vi "myRIO v1.0 Config Timer IRQ.vi"(6 "Remaining Time":u32, 7 "Timer ID":u8, 8 "error in (no error)":errorcluster, 9 "Action":enum16{"Add", "Update", "Remove"}(ring), 11 "myRIO FPGA Ref In":T2) -> (0 "error out":errorcluster, 1 "Timer IDs":u8[](array[numeric]), 3 "Callback VI Refs":T1[](array[typedef]))   [LabVIEW 2021]
uses:
  <vilib>/myRIO/Common/Instrument Driver Framework/Utilities/typedefs/Generic FPGA Reference.ctl
  <vilib>/myRIO/Common/Instrument Driver Framework/myRIO v1.0/IRQ/typedefs/Callback VI Ref.ctl
  <vilib>/myRIO/Common/Instrument Driver Framework/myRIO v1.0/IRQ/typedefs/Timer IRQ FPGA Reference.ctl
  <vilib>/myRIO/Common/Instrument Driver Framework/Utilities/typedefs/FPGA Ref Manager Action Enum.ctl
  <vilib>/Utility/error.llb/Error Cluster From Error Code.vi
  <vilib>/rvi/errors/niLvFpgaAdjustHostInterfaceError.vi
  <vilib>/rvi/interface/nirviReadWriteControl/nirviReadWriteControl.xnode
  <vilib>/rvi/interface/Simulation/niFpgaSimulationCallBeginRW.vi
  NiFpgaLv.dll
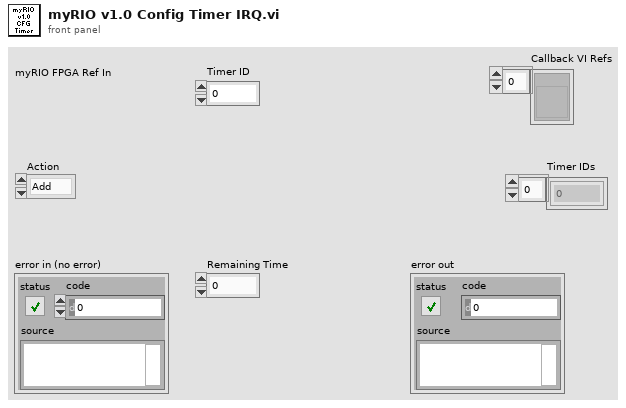
[diagram p1: front panel]
types:
  T1 = typedef "Callback VI Ref.ctl" = refnum<vi>
  T2 = typedef "Generic FPGA Reference.ctl" = refnum<k20>
  T3 = typedef "FPGA Ref Manager Action Enum.ctl" = enum16{"Get", "Set", "Reset"}
  T4 = typedef "Timer IRQ FPGA Reference.ctl" = refnum<k20>
  T5 = typedef "Timer IRQ Array.ctl" = T6[]
  T6 = typedef "Timer IRQ.ctl" = cluster{"Remaining(us)":u32, "Timer ID":u8, "Interval(us)":u32, "Callback VI Ref":T1, "Allow Overwrite?":bool, "Timer enabled?":bool}
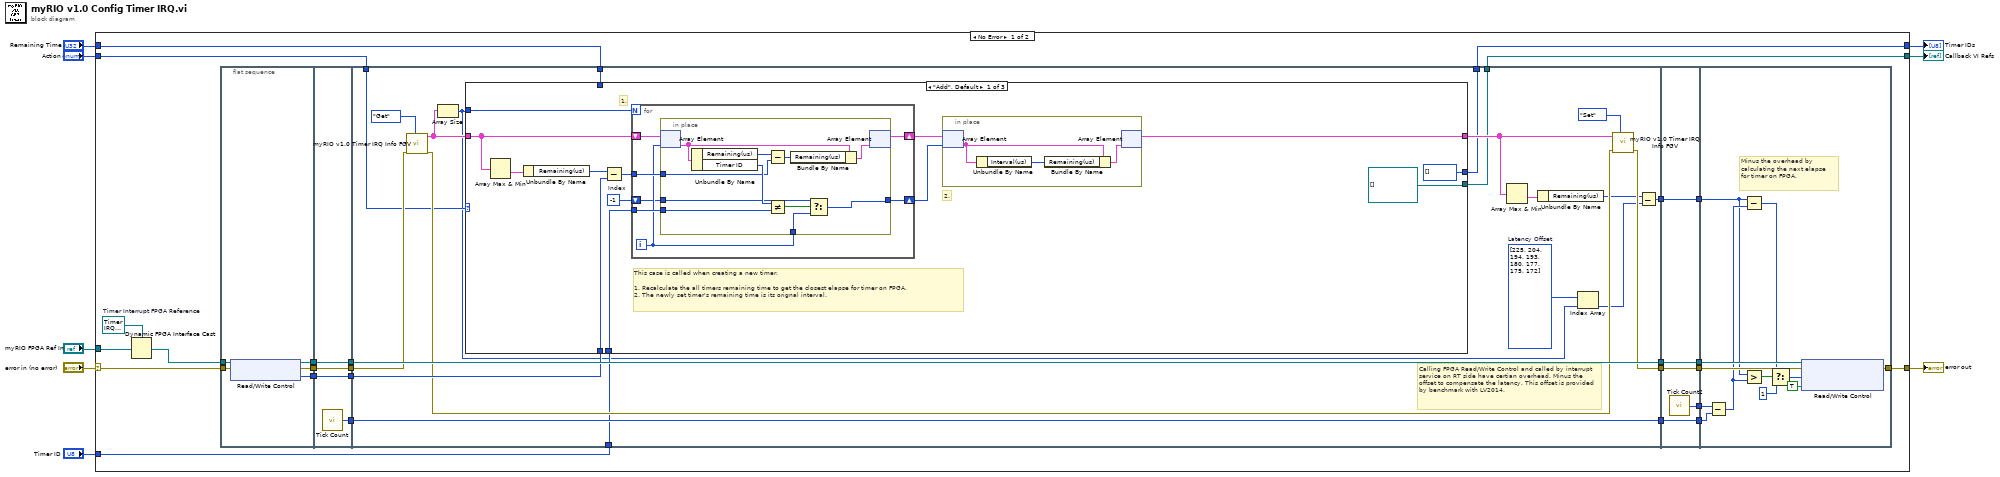
[diagram p0: block diagram]
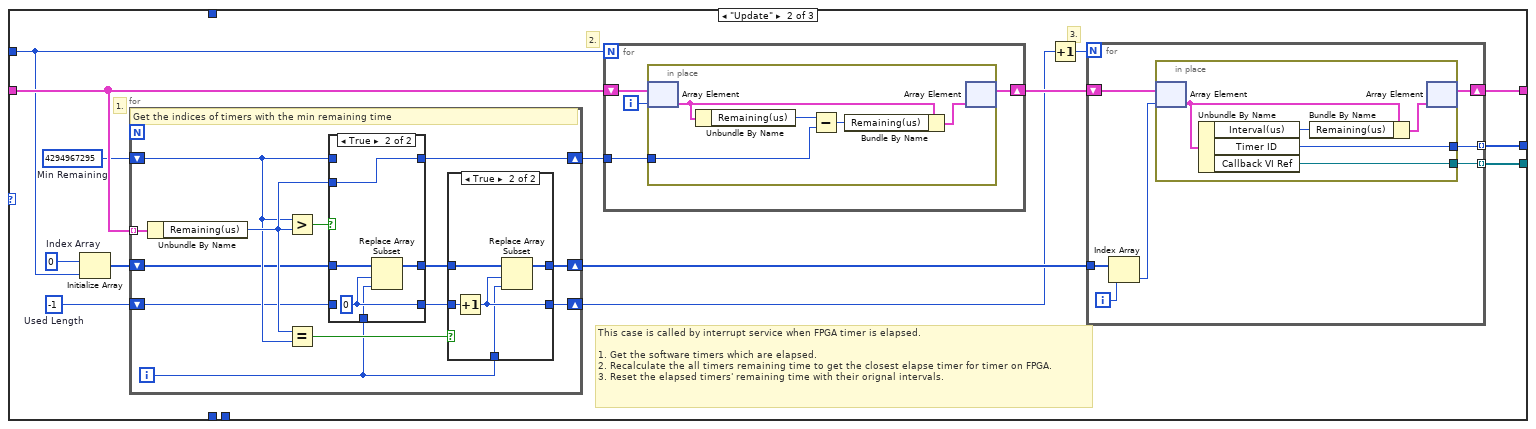
[diagram p2: hidden frame]
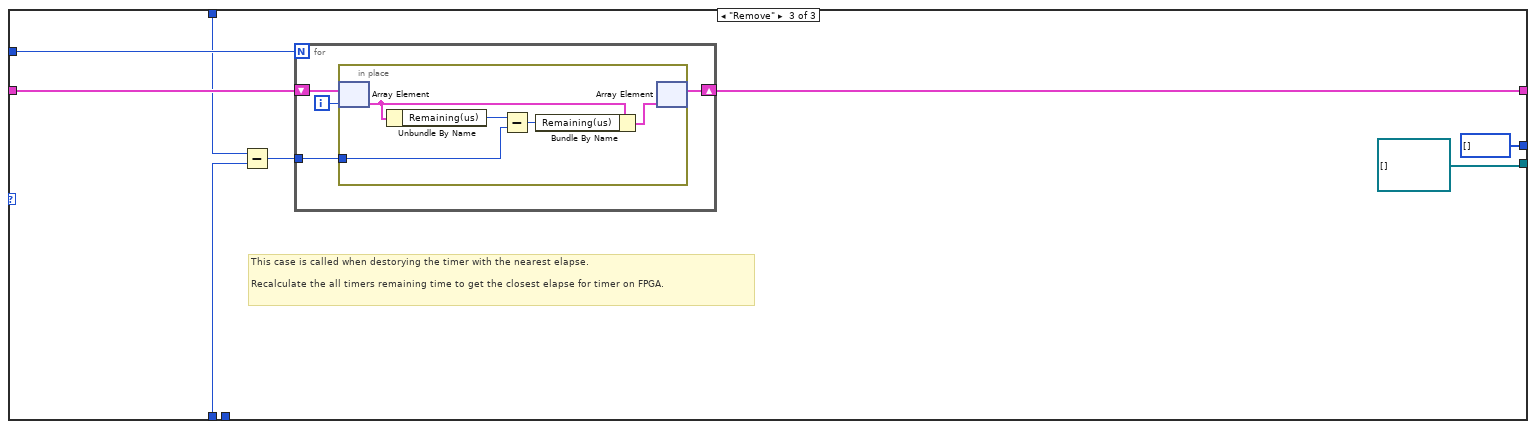
[diagram p5: hidden frame]
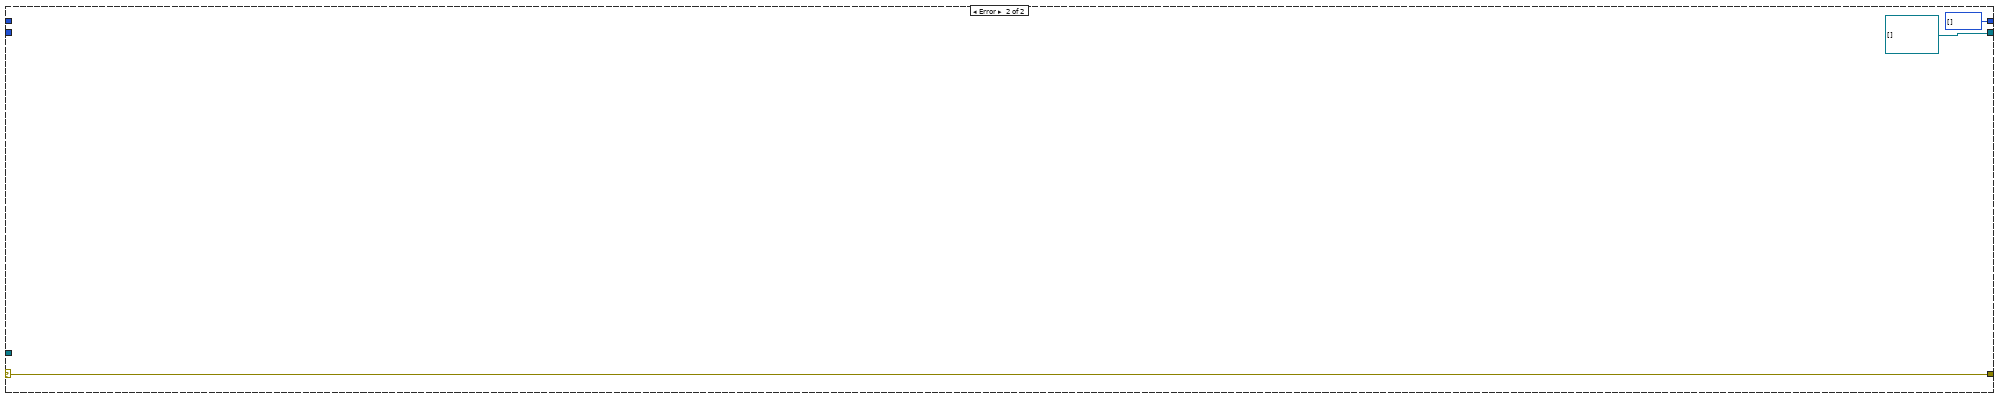
[diagram p6: hidden frame]
diagram:
  n1 = case shown="No Error" "error in (no error)" {
    selector: "error in (no error)" -> [w31 w198]
    tunnel: [w22 w198] -> w8
    tunnel: "myRIO FPGA Ref In" -> [w33 _]
    tunnel: "Timer ID" -> [w10 _]
    tunnel: [w13 T1[] []] -> w3
    tunnel: [w12 u8[] []] -> w4
    tunnel: "Action" -> [w11 _]
    tunnel: "Remaining Time" -> [w9 _]
    frame No Error {
      w34 = T4 refnum  # Timer Interrupt FPGA Reference
      n2 = Dynamic FPGA Interface Cast(Session In=w34, Type=w33) -> (Session Out=w32:T4)
      n3 = flat-sequence {
        tunnel: w32 -> [w39]
        tunnel: w31 -> [w38]
        tunnel: [w37] -> w30
        tunnel: [w36] -> w21
        tunnel: [w35] -> w16
        tunnel: w30 -> [w43]
        tunnel: [w43] -> w29
        tunnel: [w42] -> w25
        tunnel: w21 -> [w41]
        tunnel: [w41] -> w20
        tunnel: [w40] -> w17
        tunnel: w16 -> [w40]
        tunnel: w29 -> [w60]
        tunnel: [w61] -> w28
        tunnel: w25 -> [w64]
        tunnel: [w64] -> w24
        tunnel: w20 -> [w63]
        tunnel: [w63] -> w19
        tunnel: w17 -> [w62]
        tunnel: [w48] -> w15
        tunnel: [w50] -> w13
        tunnel: [w51] -> w12
        tunnel: w11 -> [w53]
        tunnel: w10 -> [w52]
        tunnel: w9 -> [w44]
        tunnel: w28 -> [w183]
        tunnel: [w183] -> w27
        tunnel: [w182] -> w26
        tunnel: w24 -> [w181]
        tunnel: [w181] -> w23
        tunnel: w19 -> [w180]
        tunnel: [w180] -> w18
        tunnel: w15 -> [w179]
        tunnel: [w179] -> w14
        tunnel: w27 -> [w193]
        tunnel: w26 -> [w195]
        tunnel: w23 -> [w194]
        tunnel: [w192] -> w22
        tunnel: w18 -> [w191]
        tunnel: w14 -> [w184]
        frame #0 {
          n4 = xnode "Read/Write Control"("FPGA VI Reference In"=w39, "error in"=w38) -> ("FPGA VI Reference Out"=w36:T4, "error out"=w37:errorcluster, "IRQ.TIMER.READ"=w35:u32)
        }
        frame #1 {
          n5 = call "Tick Count"() -> ("Tick Count(uSec)"=w42:u32)
        }
        frame #2 {
          w47 = u32[] [225, 204, 194, 193, 180, 177, 175, 172]  # Latency Offset
          # "Calling FPGA Read/Write Control and called by interrupt service on RT side have certian overhead. Minus the offset to compensate the latency. This offset is provided by benchmark with LV2014."
          n6 = call <vilib>:"myRIO v1.0 Timer IRQ Info FGV.vi"("Action"=FPGA_Ref_Manager_Action_Enum."Get", "error in (no error)"=w60) -> ("error out"=w59:errorcluster, "Timer IRQ Array out"=w56:T5)  [unwired: 8 in]
          n7 = Array Size(array=w56) -> (size(s)=w45:i32)
          n8 = case shown="\"Add\", Default" w53 {
            tunnel: w62 -> [w77 _ w169]
            tunnel: w56 -> [w70 w111 w168]
            tunnel: w45 -> [w74 w108 w166]
            tunnel: w52 -> [w73 _ _]
            tunnel: [w71 w102 w165] -> w55
            tunnel: [u8[] [] w100 u8[] []] -> w51
            tunnel: [T1[] [] w99 T1[] []] -> w50
            tunnel: w44 -> [_ _ w162]
            frame "Add", Default {
              w72 = -1  # Index
              # "2."
              # "1."
              # "This case is called when creating a new timer. \n\n1. Recalculate the all timers remaining time to get the closest elapse for timer on FPGA.\n2. The newly set timer's remaining time is its orignal interval."
              n9 = Array Max & Min(array=w70) -> (min value=w69:T6)  [unwired: 3 out]
              n10 = Unbundle By Name(w69) -> ("Remaining(us)"=w68:u32)
              n11 = Subtract(x=w68, y=w77) -> (x-y=w76:u32)
              n12 = for {
                N: w74 -> [_]
                tunnel: w73 -> [w87]
                tunnel: w76 -> [w86]
                shift-right: [w84] -> w75
                shift-left: w70 -> [w85]
                shift-right: [w82] -> w67
                shift-left: w72 -> [w81]
                i -> [w83]
                n13 = in-place {
                  in-place-border: w87 -> [w97]
                  in-place-border: w86 -> [w95]
                  in-place-border: w83 -> [w90]
                  in-place-border: [w89] -> w82
                  in-place-border: w81 -> [w88]
                  n14 = in-place-array #1(w85, w83) -> (w93:T6)
                  n15 = Unbundle By Name(w93) -> ("Remaining(us)"=w96:u32, "Timer ID"=w98:u8)
                  n16 = Subtract(x=w96, y=w95) -> (x-y=w94:u32)
                  n17 = Not Equal?(x=w98, y=w97) -> (x != y?=w91:bool)
                  n18 = Bundle By Name(cluster=w93, "Remaining(us)"=w94) -> (w92:T6)
                  n19 = Select(t=w88, s=w91, f=w90) -> (s? t:f=w89:i32)
                  n20 = in-place-array #1(w92) -> (w84:T5)  [unwired: 1 out]
                }
              }
              n21 = in-place {
                n22 = in-place-array #2(w75, w67) -> (w80:T6)
                n23 = Unbundle By Name(w80) -> ("Interval(us)"=w79:u32)
                n24 = Bundle By Name(cluster=w80, "Remaining(us)"=w79) -> (w78:T6)
                n25 = in-place-array #2(w78) -> (w71:T5)  [unwired: 1 out]
              }
            }
            frame "Update" {
              w106 = -1  # Used Length
              w109 = 0  # Index Array
              w110 = u32 4294967295  # Min Remaining
              # "3."
              # "2."
              # "1."
              # "This case is called by interrupt service when FPGA timer is elapsed. \n\n1. Get the software timers which are elapsed.\n2. Recalculate the all timers remaining time to get the closest elapse timer for timer on FPGA.\n3. Reset the elapsed timers' remaining time with their orignal intervals."
              n26 = Initialize Array(w109, w108) -> (w107:i32[])
              n27 = for {
                tunnel: w111 -> [w137] mode=indexing
                shift-right: [w135] -> w101
                shift-left: w110 -> [w133]
                shift-right: [w127] -> w105
                shift-left: w107 -> [w131]
                shift-right: [w129] -> w104
                shift-left: w106 -> [w132]
                i -> [w125]
                # "Get the indices of timers with the min remaining time"
                n28 = Unbundle By Name(w137) -> ("Remaining(us)"=w134:u32)
                n29 = Greater?(x=w133, y=w134) -> (0:w136:bool)
                n30 = Equal?(x=w134, y=w133) -> (x = y?=w130:bool)
                n31 = case shown="True" w136 {
                  tunnel: [w147 w152] -> w135
                  tunnel: w134 -> [_ w152]
                  tunnel: w133 -> [w147 _]
                  tunnel: [w146 w150] -> w128
                  tunnel: w132 -> [w146 _]
                  tunnel: w131 -> [w145 w151]
                  tunnel: w125 -> [_ w149]
                  tunnel: [w145 w148] -> w126
                  frame False {
                  }
                  frame True {
                    w150 = 0
                    n32 = Replace Array Subset(array=w151, new element=w149, index=w150) -> (w148:i32[])
                  }
                }
                n33 = case shown="True" w130 {
                  tunnel: [w139 w141] -> w129
                  tunnel: w128 -> [w139 w142]
                  tunnel: [w138 w143] -> w127
                  tunnel: w126 -> [w138 w144]
                  tunnel: w125 -> [_ w140]
                  frame False {
                  }
                  frame True {
                    n34 = Increment(x=w142) -> (x+1=w141:i32)
                    n35 = Replace Array Subset(array=w144, new element=w140, index=w141) -> (w143:i32[])
                  }
                }
              }
              n36 = for {
                N: w108 -> [_]
                tunnel: w101 -> [w156]
                shift-right: [w154] -> w112
                shift-left: w111 -> [w155]
                i -> [w153]
                n37 = in-place {
                  in-place-border: w156 -> [w160]
                  n38 = in-place-array #3(w155, w153) -> (w158:T6)
                  n39 = Unbundle By Name(w158) -> ("Remaining(us)"=w161:u32)
                  n40 = Subtract(x=w161, y=w160) -> (x-y=w159:u32)
                  n41 = Bundle By Name(cluster=w158, "Remaining(us)"=w159) -> (w157:T6)
                  n42 = in-place-array #3(w157) -> (w154:T5)  [unwired: 1 out]
                }
              }
              n43 = Increment(x=w104) -> (x+1=w103:i32)
              n44 = for {
                N: w103 -> [_]
                shift-right: [w119] -> w102
                shift-left: w112 -> [w118]
                tunnel: w105 -> [w117]
                tunnel: [w114] -> w100 mode=indexing
                tunnel: [w113] -> w99 mode=indexing
                i -> [w116]
                n45 = Index Array(array=w117, index=w116) -> (element=w115:i32)
                n46 = in-place {
                  in-place-border: [w121] -> w114
                  in-place-border: [w120] -> w113
                  n47 = in-place-array #4(w118, w115) -> (w124:T6)
                  n48 = Unbundle By Name(w124) -> ("Interval(us)"=w123:u32, "Timer ID"=w121:u8, "Callback VI Ref"=w120:T1)
                  n49 = Bundle By Name(cluster=w124, "Remaining(us)"=w123) -> (w122:T6)
                  n50 = in-place-array #4(w122) -> (w119:T5)  [unwired: 1 out]
                }
              }
            }
            frame "Remove" {
              # "This case is called when destorying the timer with the nearest elapse. \n\nRecalculate the all timers remaining time to get the closest elapse for timer on FPGA."
              n51 = Subtract(x=w162, y=w169) -> (x-y=w167:u32)
              n52 = for {
                N: w166 -> [_]
                tunnel: w167 -> [w173]
                shift-right: [w171] -> w165
                shift-left: w168 -> [w172]
                i -> [w170]
                n53 = in-place {
                  in-place-border: w173 -> [w177]
                  n54 = in-place-array #5(w172, w170) -> (w175:T6)
                  n55 = Unbundle By Name(w175) -> ("Remaining(us)"=w178:u32)
                  n56 = Subtract(x=w178, y=w177) -> (x-y=w176:u32)
                  n57 = Bundle By Name(cluster=w175, "Remaining(us)"=w176) -> (w174:T6)
                  n58 = in-place-array #5(w174) -> (w171:T5)  [unwired: 1 out]
                }
              }
            }
          }
          n59 = Array Max & Min(array=w55) -> (min value=w54:T6)  [unwired: 3 out]
          n60 = Unbundle By Name(w54) -> ("Remaining(us)"=w49:u32)
          n61 = Index Array(array=w47, index=w45) -> (element=w46:u32)
          n62 = call <vilib>:"myRIO v1.0 Timer IRQ Info FGV.vi"("Action"=FPGA_Ref_Manager_Action_Enum."Set", "error in (no error)"=w59, "Timer IRQ Array in"=w55) -> ("error out"=w61:errorcluster)  [unwired: 7 in, 1 out]
          n63 = Subtract(x=w49, y=w46) -> (x-y=w48:u32)
        }
        frame #3 {
          n64 = call "Tick Count2"() -> ("Tick Count(uSec)"=w182:u32)
        }
        frame #4 {
          # "Minus the overhead by calculating the next elapse for timer on FPGA."
          n65 = Subtract(x=w195, y=w194) -> (x-y=w189:u32)
          n66 = Subtract(x=w184, y=w189) -> (x-y=w187:u32)
          n67 = Greater?(x=w184, y=w189) -> (0:w188:bool)
          n68 = Select(t=w187, s=w188, f=u32 1) -> (s? t:f=w186:u32)
          n69 = xnode "Read/Write Control"("FPGA VI Reference In"=w191, "error in"=w193, "IRQ.TIMER.WRITE"=w186, "IRQ.TIMER.SETTIME"=TRUE ("TIMER.SetTime")) -> ("error out"=w192:errorcluster)  [unwired: 1 out]
        }
      }
    }
    frame Error {
    }
  }
  "error out" <- w8
  "Callback VI Refs" <- w3
  "Timer IDs" <- w4
